vi "VI Tree.vi"   [LabVIEW 2016, in "Agilent 4263X.lvlib"]
doc: "This is the instrument driver for the Agilent 4263A/B. The VI Tree displays all the user-callable VIs of the instrument driver in an organized table."
uses:
  <instrlib>/Agilent 4263X/Agilent 4263X.lvlib
panel:
  # "(c) 2015 <National Instruments>.  ALL RIGHTS RESERVED."
  # "See Diagram Box\nfor VI Tree"
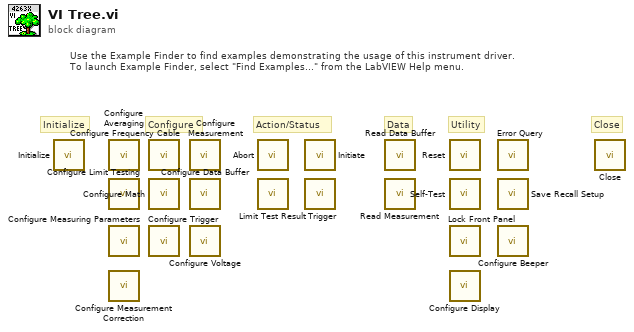
[diagram p0: block diagram]
diagram:
  # "Utility"
  # "Data"
  # "Action/Status"
  # "Configure"
  # "Close"
  # "Initialize"
  # "Use the Example Finder to find examples demonstrating the usage of this instrument driver.\nTo launch Example Finder, select \"Find Examples...\" from the LabVIEW Help menu."
  n1 = call <instrlib>:"Initialize.vi"() -> ()  [unwired: 10 in, 2 out]
  n2 = call <instrlib>:"Configure Averaging.vi"() -> ()  [unwired: 10 in, 2 out]
  n3 = call <instrlib>:"Configure Limit Testing.vi"() -> ()  [unwired: 14 in, 2 out]
  n4 = call <instrlib>:"Configure Measuring Parameters.vi"() -> ()  [unwired: 14 in, 2 out]
  n5 = call <instrlib>:"Configure Measurement Correction.vi"() -> ()  [unwired: 14 in, 2 out]
  n6 = call <instrlib>:"Configure Frequency Cable.vi"() -> ()  [unwired: 14 in, 2 out]
  n7 = call <instrlib>:"Configure Math.vi"() -> ()  [unwired: 14 in, 2 out]
  n8 = call <instrlib>:"Configure Trigger.vi"() -> ()  [unwired: 10 in, 2 out]
  n9 = call <instrlib>:"Configure Measurement.vi"() -> ()  [unwired: 10 in, 2 out]
  n10 = call <instrlib>:"Configure Data Buffer.vi"() -> ()  [unwired: 14 in, 2 out]
  n11 = call <instrlib>:"Configure Voltage.vi"() -> ()  [unwired: 14 in, 2 out]
  n12 = call <instrlib>:"Abort.vi"() -> ()  [unwired: 10 in, 2 out]
  n13 = call <instrlib>:"Limit Test Result.vi"() -> ()  [unwired: 9 in, 3 out]
  n14 = call <instrlib>:"Initiate.vi"() -> ()  [unwired: 10 in, 2 out]
  n15 = call <instrlib>:"Trigger.vi"() -> ()  [unwired: 10 in, 2 out]
  n16 = call <instrlib>:"Read Data Buffer.vi"() -> ()  [unwired: 9 in, 3 out]
  n17 = call <instrlib>:"Read Measurement.vi"() -> ()  [unwired: 9 in, 7 out]
  n18 = call <instrlib>:"Reset.vi"() -> ()  [unwired: 10 in, 2 out]
  n19 = call <instrlib>:"Self-Test.vi"() -> ()  [unwired: 8 in, 4 out]
  n20 = call <instrlib>:"Lock Front Panel.vi"() -> ()  [unwired: 10 in, 2 out]
  n21 = call <instrlib>:"Configure Display.vi"() -> ()  [unwired: 10 in, 2 out]
  n22 = call <instrlib>:"Error Query.vi"() -> ()  [unwired: 8 in, 4 out]
  n23 = call <instrlib>:"Save Recall Setup.vi"() -> ()  [unwired: 10 in, 2 out]
  n24 = call <instrlib>:"Configure Beeper.vi"() -> ()  [unwired: 10 in, 2 out]
  n25 = call <instrlib>:"Close.vi"() -> ()  [unwired: 11 in, 1 out]
